vi "Create with Path.vi"(7 "Existing FlexWorktable":refnum<class "FlexWorktable.lvclass">, 8 "error in (no error)":errorcluster, 10 "prefix":string, 11 "flex_config path":path) -> (0 "error out":errorcluster, 3 "FlexWorktable out":refnum<class "FlexWorktable.lvclass">)   [LabVIEW 2017, in "FlexWorktable.lvclass"]
uses:
  FlexWorktable.lvclass
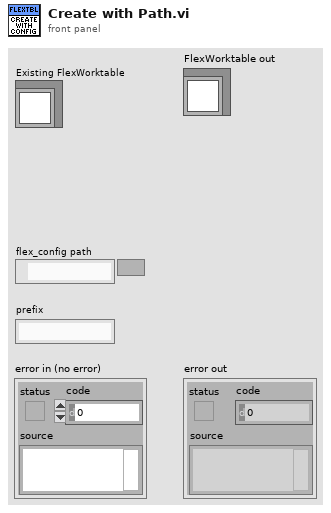
[diagram p1: front panel]
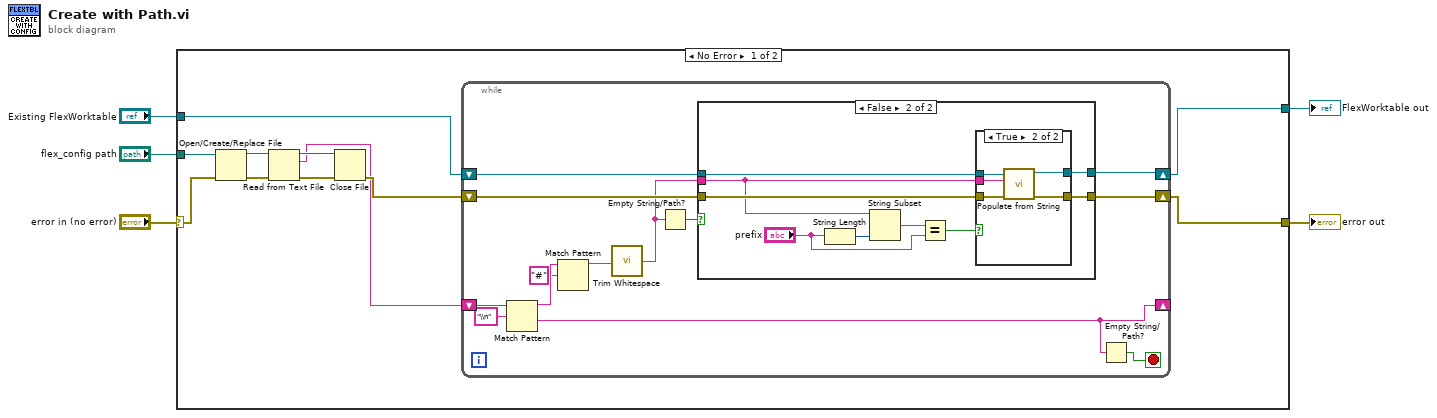
[diagram p0: block diagram]
diagram:
  n1 = case shown="No Error" "error in (no error)" {
    selector: "error in (no error)" -> [w10 w48]
    tunnel: [w8 w48] -> w4
    tunnel: [w7 _] -> w3
    tunnel: "flex_config path" -> [w9 _]
    tunnel: "Existing FlexWorktable" -> [w6 _]
    frame No Error {
      n2 = Open/Create/Replace File(file path (use dialog)=w9, error in=w10) -> (refnum out=w16:refnum<file>, error out=w15:errorcluster)  [unwired: 4 in, 1 out]
      n3 = Read from Text File(file (use dialog)=w16, error in=w15) -> (refnum out=w14:refnum<file>, text=w11:string, error out=w13:errorcluster)  [unwired: 2 in, 1 out]
      n4 = Close File(refnum=w14, error in=w13) -> (error out=w12:errorcluster)  [unwired: 1 out]
      n5 = while {
        shift-right: [w28] -> _
        shift-left: w11 -> [w29]
        shift-right: [w25] -> w7
        shift-left: w6 -> [w26]
        shift-right: [w23] -> w8
        shift-left: w12 -> [w24]
        stop <- w27 stop-if-true
        n6 = Match Pattern(string=w29, regular expression="\\n") -> (before substring=w20:string, after substring=w28:string)  [unwired: 1 in, 2 out]
        n7 = Match Pattern(string=w20, regular expression="#") -> (before substring=w18:string)  [unwired: 1 in, 3 out]
        n8 = call <vilib>:"Trim Whitespace.vi"("string"=w18) -> ("trimmed string"=w17:string)  [unwired: 1 in]
        n9 = Empty String/Path?(string/path=w17) -> (empty?=w21:bool)
        n10 = case shown="False" w21 {
          tunnel: w26 -> [w31 w40]
          tunnel: [w31 w39] -> w25
          tunnel: w24 -> [w30 w38]
          tunnel: w17 -> [_ w35]
          tunnel: [w30 w37] -> w23
          frame True {
          }
          frame False {
            n11 = String Length(string="prefix") -> (length=w36:i32)
            n12 = String Subset(string=w35, length (rest)=w36) -> (substring=w34:string)  [unwired: 1 in]
            n13 = Equal?(x=w34, y="prefix") -> (x = y?=w32:bool)
            n14 = case shown="True" w32 {
              tunnel: w40 -> [w42 w47]
              tunnel: [w42 w46] -> w39
              tunnel: w38 -> [w41 w45]
              tunnel: [w41 w44] -> w37
              tunnel: w35 -> [_ w43]
              frame False {
              }
              frame True {
                n15 = call-dynamic "Populate from String.vi"("error in (no error)"=w45, "Line in"=w43, "FlexWorktable in"=w47) -> ("error out"=w44:errorcluster, "FlexWorktable out"=w46:refnum<class "FlexWorktable.lvclass">)  [unwired: 7 in]
              }
            }
          }
        }
        n16 = Empty String/Path?(string/path=w28) -> (empty?=w27:bool)
      }
    }
    frame Error {
    }
  }
  "error out" <- w4
  "FlexWorktable out" <- w3
